vi "polish_instrument_command.vi"(8 "error in (no error)":errorcluster, 11 "Instrument Command In":string="TRIGger:AND:ENABle {{ON | 1} | {OFF | 0}} ") -> (0 "error out":errorcluster, 3 "Instrument Command Out":string)   [LabVIEW 2018]
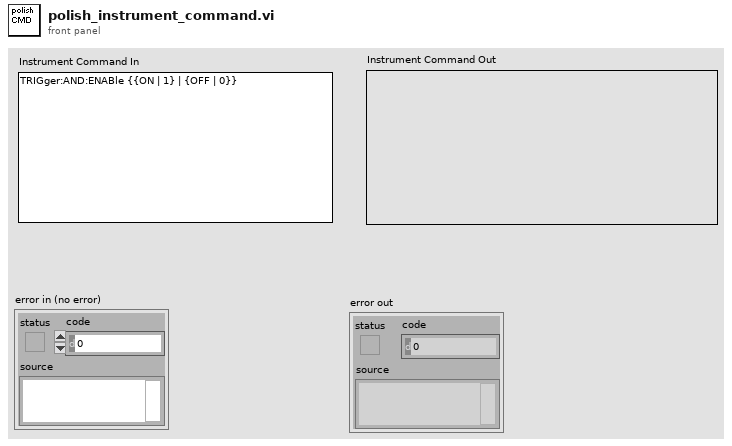
[diagram p1: front panel]
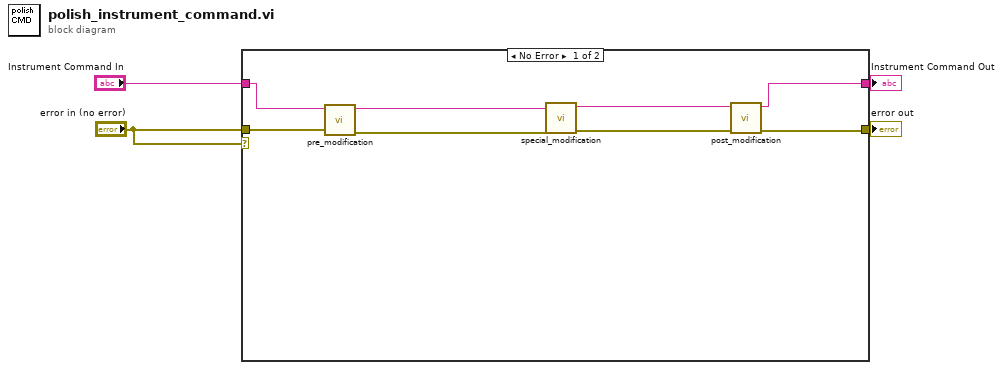
[diagram p0: block diagram]
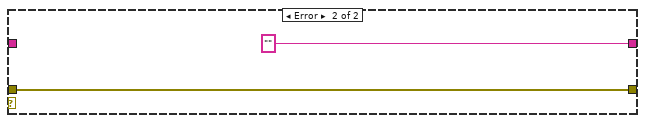
[diagram p2: hidden frame]
diagram:
  n1 = case shown="No Error" "error in (no error)" {
    tunnel: [w10 "" ("result string")] -> w4
    tunnel: "Instrument Command In" -> [w12 _]
    tunnel: "error in (no error)" -> [w11 w13]
    tunnel: [w9 w13] -> w1
    frame No Error {
      n2 = call "pre_modification.vi"("error in (no error)"=w11, "Instrument Command In"=w12) -> ("error out"=w7:errorcluster, "Instrument Command Out"=w8:string)  [unwired: 8 out]
      n3 = call "special_modification.vi"("error in"=w7, "Instrument Command In"=w8) -> ("error out"=w6:errorcluster, "Instrument Command Out"=w5:string)  [unwired: 8 out]
      n4 = call "post_modification.vi"("error in"=w6, "Instrument Command In"=w5) -> ("error out"=w9:errorcluster, "Instrument Command Out"=w10:string)  [unwired: 8 out]
    }
    frame Error {
    }
  }
  "Instrument Command Out" <- w4
  "error out" <- w1
